vi "stoperaseDOLT_img.vi"   [LabVIEW 2013]
types:
  T1 = cluster{"DOLT":refnum<k21>, "E_DOLT":errorcluster}
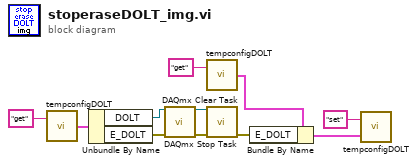
[diagram p0: block diagram]
diagram:
  n1 = call "tempconfigDOLT.vi"("command"="get") -> ("Temp Config out"=w10:T1)  [unwired: 1 in]
  n2 = Unbundle By Name(w10) -> ("DOLT"=w9:refnum<k21>, "E_DOLT"=w8:errorcluster)
  n3 = call <vilib>:"DAQmx Stop Task.vi"("task/channels in"=w9, "error in"=w8) -> ("task out"=w7:refnum<k21>, "error out"=w6:errorcluster)  [unwired: 12 in]
  n4 = call "tempconfigDOLT.vi"("command"="get") -> ("Temp Config out"=w3:T1)  [unwired: 1 in]
  n5 = call <vilib>:"DAQmx Clear Task.vi"("task in"=w7, "error in"=w6) -> ("error out"=w5:errorcluster)  [unwired: 13 in]
  n6 = Bundle By Name(cluster=w3, "E_DOLT"=w5) -> (w1:T1)
  n7 = call "tempconfigDOLT.vi"("Temp Config in"=w1, "command"="set") -> ()  [unwired: 1 out]
